vi "Trim String.vi"(1 "inStr":string caption="In String") -> (0 "outStr":string caption="Out String")   [LabVIEW 2015]
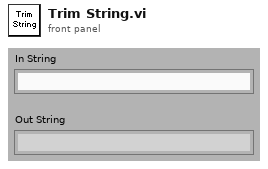
[diagram p1: front panel]
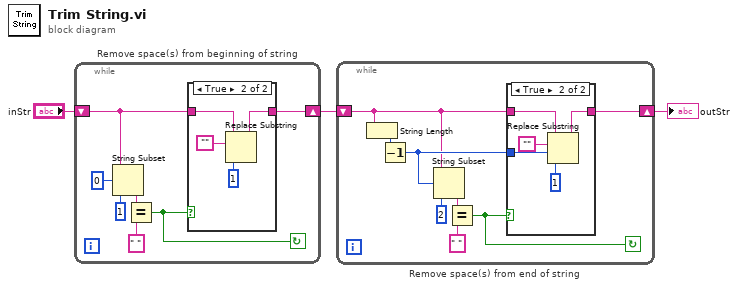
[diagram p0: block diagram]
diagram:
  n1 = while "Remove space(s) from beginning of string" {
    shift-left: "inStr" -> [w5]
    shift-right: [w8] -> w2
    stop <- w7 continue-if-true
    n2 = String Subset(string=w5, offset (0)=0, length (rest)=1 ("length (rest)")) -> (substring=w6:string)
    n3 = Equal?(x=w6, y=" ") -> (x = y?=w7:bool)
    n4 = case shown="True" w7 {
      tunnel: w5 -> [w11 w15]
      tunnel: [w11 w13] -> w8
      frame False {
      }
      frame True {
        n5 = Replace Substring(2:1 ("length (len. of substring)"), 4:"" ("Empty String Constant"), 5:w15) -> (1:w13:string)  [unwired: 2 out]
      }
    }
  }
  n6 = while "Remove space(s) from end of string" {
    shift-left: w2 -> [w16]
    shift-right: [w23] -> w1
    stop <- w22 continue-if-true
    n7 = String Length(string=w16) -> (length=w19:i32)
    n8 = Decrement(x=w19) -> (x-1=w17:i32)
    n9 = String Subset(string=w16, offset (0)=w17, length (rest)=2 ("length (rest)")) -> (substring=w21:string)
    n10 = Equal?(x=w21, y=" ") -> (x = y?=w22:bool)
    n11 = case shown="True" w22 {
      tunnel: w16 -> [w24 w27]
      tunnel: [w24 w28] -> w23
      tunnel: w17 -> [_ w25]
      frame False {
      }
      frame True {
        n12 = Replace Substring(2:1 ("length (len. of substring)"), 3:w25, 4:"", 5:w27) -> (1:w28:string)  [unwired: 1 out]
      }
    }
  }
  "outStr" <- w1
